vi "DBL to Matlab String.vi"(8 "error in (no error)":errorcluster, 10 "Value":dbl, 11 "Variable name":string) -> (0 "error out":errorcluster, 3 "String":string)   [LabVIEW 2011, in "Matlab API.lvlib"]
uses:
  Matlab API.lvlib
panel:
  out "Array":u8[](array[numeric]) format="%x"
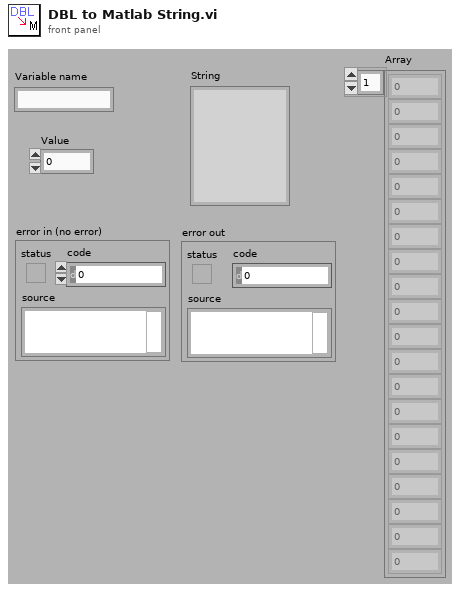
[diagram p1: front panel]
types:
  T1 = enum16{"big-endian, network order", "native, host order", "little-endian"}
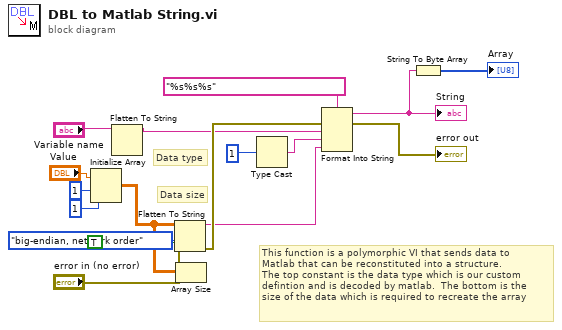
[diagram p0: block diagram]
diagram:
  # "Data size"
  # "Data type"
  # "This function is a polymorphic VI that sends data to\nMatlab that can be reconstituted into a structure.\nThe top constant is the data type which is our custom\ndefintion and is decoded by matlab.  The bottom is the\nsize of the data which is required to recreate the array"
  n1 = Initialize Array("Value", 1 ("dimension size"), 1 ("dimension size")) -> (w1:dbl[][])
  n2 = Flatten To String(anything="Variable name") -> (data string=w8:string)  [unwired: 1 in, 4 out]
  n3 = Flatten To String(anything=w1, prepend array or string size? (T)=TRUE, byte order (0:big-endian, network order)=T1."big-endian, network order", error in (no error)="error in (no error)") -> (data string=w5:string, error out=w14:errorcluster)  [unwired: 1 out]
  n4 = Array Size(array=w1) -> ()  [unwired: 1 out]
  n5 = Type Cast(x=1 ("input 2")) -> (*(type *) &x=w10:string)  [unwired: 1 out]
  n6 = Format Into String(format string="%s%s%s", error in=w14, w8, w10, w5) -> (resulting string=w11:string, error out=→"error out":errorcluster)  [unwired: 1 in]
  "String" <- w11
  n7 = String To Byte Array(string=w11) -> (unsigned byte array=→"Array":u8[])
